vi "Get credit available.vi"(8 "error in (no error)":errorcluster, 10 "Credito Disponible":dbl, 11 "Paquetes Disonibles in":refnum<class "Paquetes Disonibles.lvclass">) -> (0 "error out":errorcluster, 3 "Paquetes Disonibles out":refnum<class "Paquetes Disonibles.lvclass">)   [LabVIEW 2021, in "Paquetes Disonibles.lvlib" / "Paquetes Disonibles.lvclass"]
uses:
  Paquetes Disonibles.lvclass
  Paquetes Disonibles.lvclass/Paquetes Disonibles.ctl
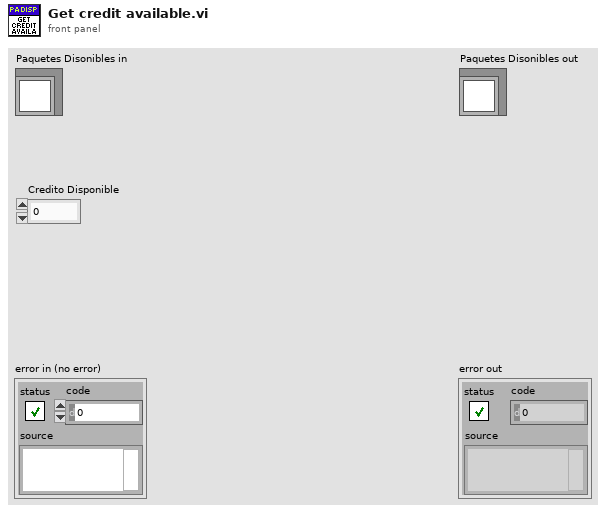
[diagram p1: front panel]
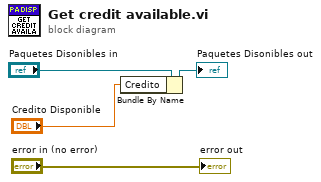
[diagram p0: block diagram]
diagram:
  n1 = Bundle By Name(cluster="Paquetes Disonibles in", "Credito"="Credito Disponible") -> (→"Paquetes Disonibles out":refnum<class "Paquetes Disonibles.lvclass">)
  "error out" <- "error in (no error)"
